vi "test图层-修改中.vi"() -> ()   [LabVIEW 2018]
doc: "This example demonstrates the use of binary morphological reconstruction in the particle analysis. The example allows you to keep the particles completely inside the ROI, completely outside the ROI or on the ROI."
uses:
  <vilib>/vision/NI_Vision_Development_Module.lvlib
panel:
  out "下":i32
  out "右":i32
  out "上":i32
  out "左":i32
  out "面积":i32
  out "标准差":sgl
  out "平均值":sgl
  out "最大灰度值":sgl
  out "最小灰度值":sgl
  out "选中框灰度表":u32[](graph)
  out "Image Dst Out":T1(plugin-control)
  out "全图灰度级信息":T2 {"标准差" format="%.2f"; "均值" format="%.2f"; "相邻灰度级间隔" format="%.2f"; "起始灰度值" format="%.2f"; "最大值" format="%.2f"; "最小值" format="%.2f"}
  out "图片灰度表":u32[](graph)
  in  "Font, Size & Style 2":T3={"Desired Font (Application)"=enum."Application Font", "[User-specified Font]"={"Font Name"="", "Size"=12, "Strikeout?"=FALSE, "Italic?"=FALSE, "Underline?"=FALSE, "Outline?"=FALSE, "Shadow?"=FALSE, "Bold?"=FALSE, "Rotation Angle"=0.0}, "Horizontal Alignment"=0, "Vertical Alignment"=0} {"Vertical Alignment" items=["Bottom", "Top", "Baseline"]; "Horizontal Alignment" items=["Left", "Center", "Right"]; "[User-specified Font]"."Rotation Angle" format="%.2f"}
  in  "选择框号":bool
  out "当前选择框的编号":dbl
  out "框总数":dbl
  in  "Font, Size & Style":T3={"Desired Font (Application)"=enum."Application Font", "[User-specified Font]"={"Font Name"="", "Size"=12, "Strikeout?"=FALSE, "Italic?"=FALSE, "Underline?"=FALSE, "Outline?"=FALSE, "Shadow?"=FALSE, "Bold?"=FALSE, "Rotation Angle"=0.0}, "Horizontal Alignment"=0, "Vertical Alignment"=0} {"Vertical Alignment" items=["Bottom", "Top", "Baseline"]; "Horizontal Alignment" items=["Left", "Center", "Right"]; "[User-specified Font]"."Rotation Angle" format="%.2f"}
  out "框组":T4(array[cluster])
  in  "单次删除":bool
  in  "Operation":enum16{"overlay rectangle"}(ring)
  out "标注图":T1(plugin-control)
  in  "退出标注":bool
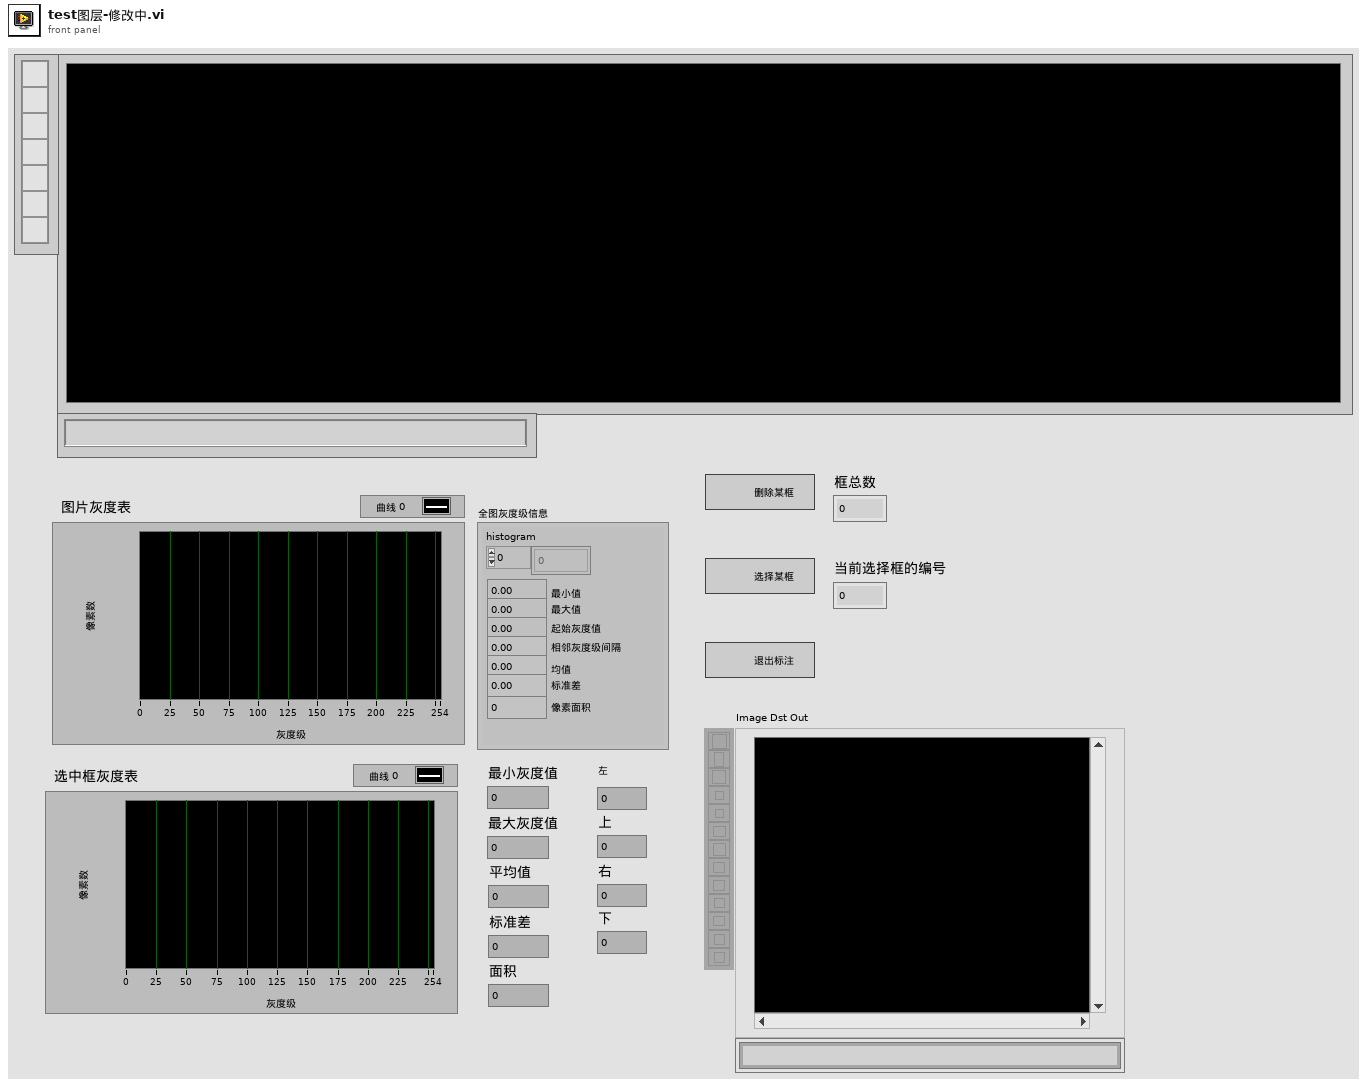
[diagram p1: front panel]
types:
  T1 = typedef "IMAQ Image.ctl" = refnum<image>
  T2 = cluster{"histogram":u32[], "最小值":sgl, "最大值":sgl, "起始灰度值":sgl, "相邻灰度级间隔":sgl, "均值":sgl, "标准差":sgl, "像素面积":i32}
  T3 = cluster{"Desired Font (Application)":enum16{"User-specified Font", "Application Font", "System Font", "Dialog Font"}, "[User-specified Font]":cluster{"Font Name":string, "Size":i16, "Strikeout?":bool, "Italic?":bool, "Underline?":bool, "Outline?":bool, "Shadow?":bool, "Bold?":bool, "Rotation Angle":dbl}, "Horizontal Alignment":i16, "Vertical Alignment":i16}
  T4 = cluster{"Global Rectangle":i32[], "Contours":cluster{"Contour Type":u32, "ROI Type":u32, "Points":i32[]}[]}[]
  T5 = typedef "Image Type" = u32
  T6 = cluster{"Global Rectangle":i32[], "Contours":cluster{"Contour Type":u32, "ROI Type":u32, "Points":i32[]}[]}
  T7 = typedef "IMAQ Rectangle" = cluster{"Left":i32, "Top":i32, "Right":i32, "Bottom":i32, "Rotation":dbl}
  T8 = cluster{"histogram":u32[], "Minimal Value":sgl, "Maximal Value":sgl, "Starting Value":sgl, "Interval Width":sgl, "Mean Value":sgl, "Standard  Variation":sgl, "Area (pixels)":i32}
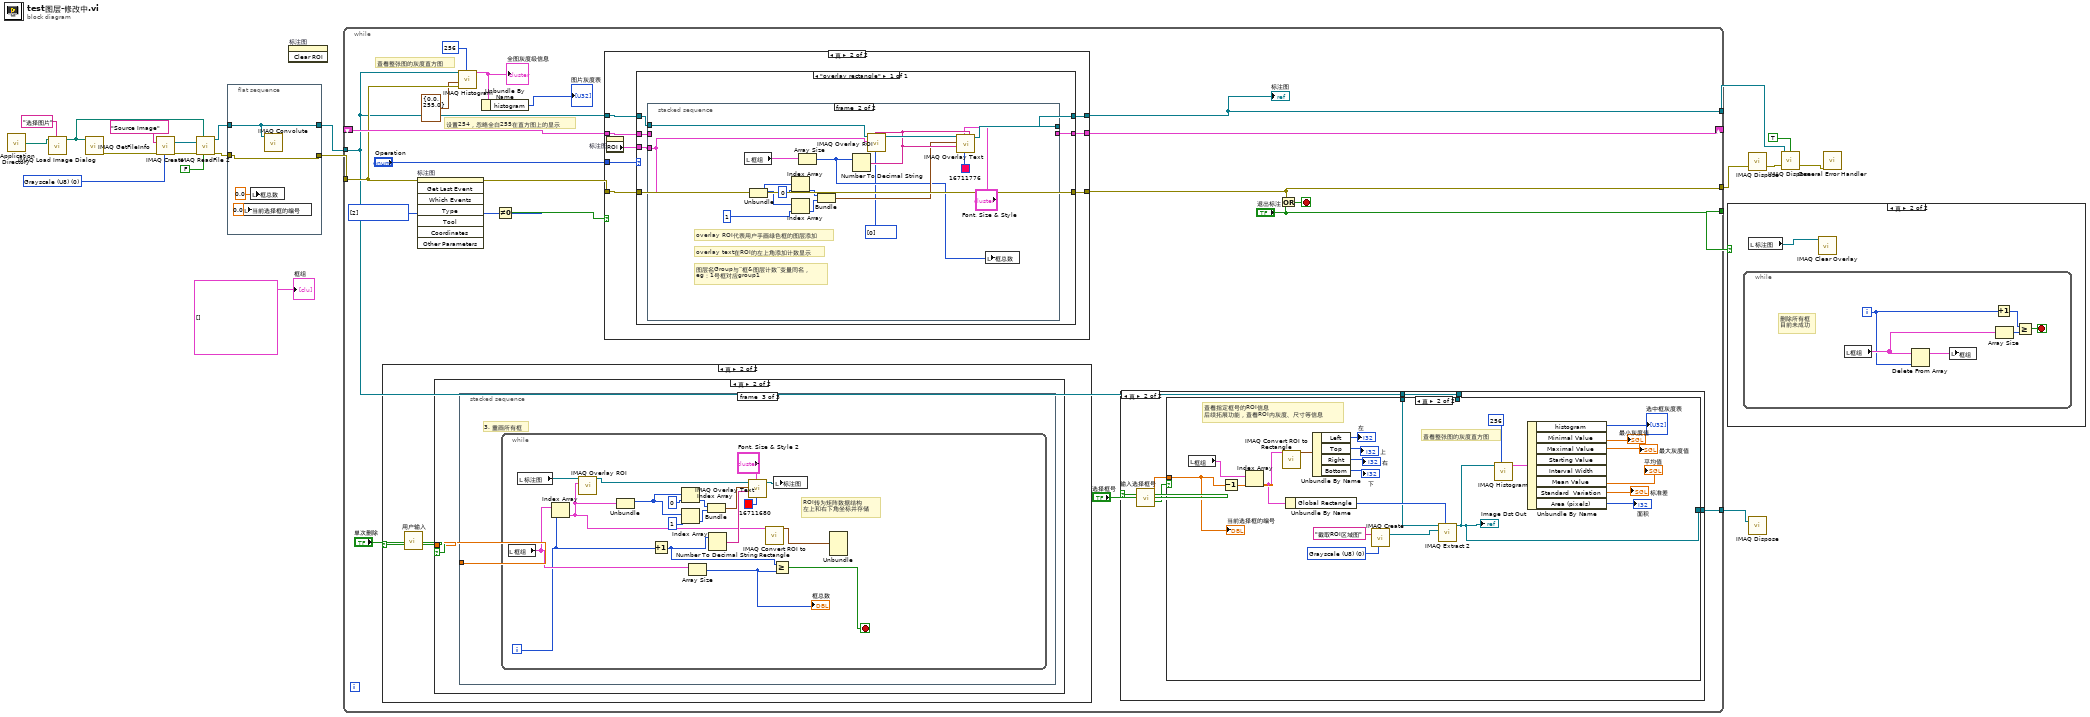
[diagram p0: block diagram]
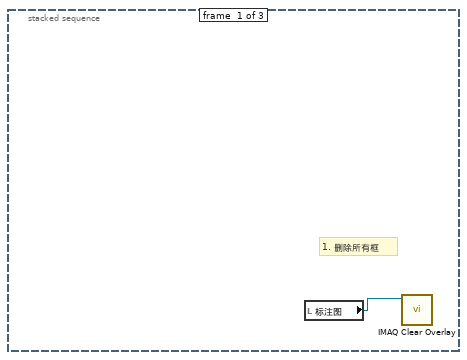
[diagram p7: hidden frame]
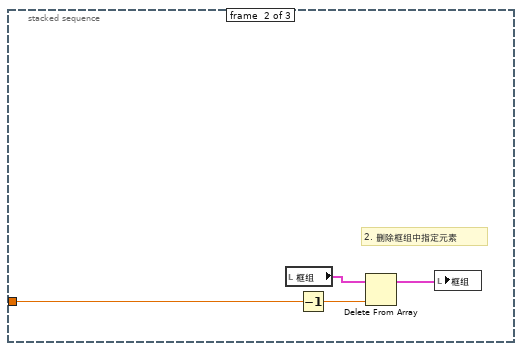
[diagram p8: hidden frame]
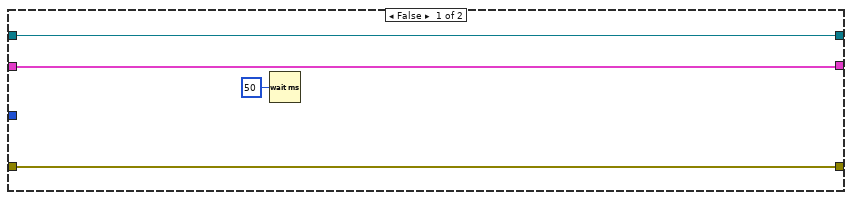
[diagram p9: hidden frame]
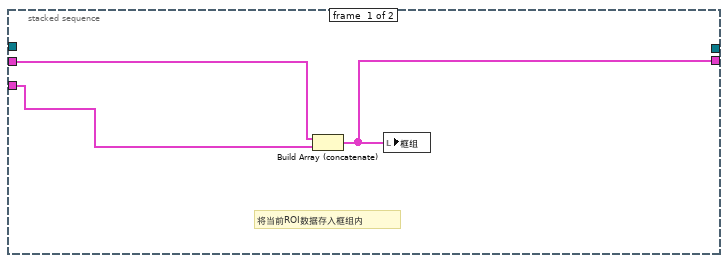
[diagram p10: hidden frame]
diagram:
  w12 = T5 0 items=["Grayscale (U8)", "Grayscale (I16)", "Grayscale (SGL)", "Complex (CSG)", "RGB (U32)", "HSL (U32)", "RGB (U64)", "Grayscale (U16)"] ("Image Type")
  n1 = call <vilib>:"Application Directory.vi"() -> ("Application Directory"=w13:path)
  n2 = call "IMAQ Load Image Dialog"("Prompt"="选择图片" ("prompt"), "Start Path"=w13) -> ("Path"=w19:path)  [unwired: 7 in, 2 out]
  n3 = call "IMAQ GetFileInfo"("File Path"=w19) -> ("error out"=w17:errorcluster)  [unwired: 4 in, 6 out]
  n4 = call "IMAQ Create"("Image Name"="Source Image", "Image Type"=w12, "error in (no error)"=w17) -> ("New Image"=w15:T1, "error out"=w14:errorcluster)  [unwired: 2 in]
  n5 = call "IMAQ ReadFile 2"("Use File Path Image Type"=FALSE, "File Path"=w19, "error in (no error)"=w14, "Image"=w15) -> ("error out"=w4:errorcluster, "Image Out"=w2:T1)  [unwired: 3 in, 3 out]
  n6 = flat-sequence {
    tunnel: [w23] -> w3
    tunnel: w4 -> [w23]
    tunnel: w2 -> [w22]
    tunnel: [w22] -> w1
    frame #0 {
      n7 = local write "当前选择框的编号"(0.0 ("当前框的编号")) -> ()
      n8 = local write "框总数"(0.0 ("框总数")) -> ()
      n9 = call "IMAQ Convolute"("Image Src"=w22) -> ()  [unwired: 9 in, 2 out]
    }
  }
  n10 = invoke on="标注图" class="ImageControl" method="Clear ROI"() -> ()  [unwired: 3 in, 3 out]
  n11 = while {
    tunnel: [w28] -> w10
    tunnel: [w41] -> w8
    shift-right: [w37] -> _
    shift-left: _ -> [w36]
    tunnel: ["退出标注"] -> w20
    tunnel: w3 -> [w33]
    tunnel: [w27] -> w5
    tunnel: w1 -> [w26]
    stop <- w40 stop-if-true
    w43 = i32[] [2] items=["No Event"=0, "Click Event"=1, "Draw Event"=2, "Size Event"=4, "Scroll Event"=5, "Double Click Event"=8] ("Which Events")
    # "设置254，忽略全白255在直方图上的显示"
    # "查看整张图的灰度直方图"
    n12 = case shown="真" "单次删除" {
      frame False {
      }
      frame True {
        n13 = call "用户输入"() -> ("框号"=w76:dbl, "确定"=w77:bool)  [unwired: 17 in, 1 out]
        n14 = case shown="真" w77 {
          tunnel: w76 -> [_ w78]
          frame False {
            # "用户取消操作"
          }
          frame True {
            n15 = stacked-sequence {
              tunnel: w78 -> [_ w82 _]
              frame #0 {
                # "1. 删除所有框"
                n16 = local read "标注图"() -> (w79:T1)
                n17 = call "IMAQ Clear Overlay"("Image"=w79) -> ()  [unwired: 9 in, 2 out]
              }
              frame #1 {
                # "2. 删除框组中指定元素"
                n18 = local read "框组"() -> (w83:T4)
                n19 = Decrement(x=w82) -> (x-1=w81:dbl)
                n20 = Delete From Array(array=w83, index=w81) -> (array with subset deleted=w80:T4)  [unwired: 1 in, 1 out]
                n21 = local write "框组"(w80) -> ()
              }
              frame #2 {
                # "3. 重画所有框"
                n22 = while {
                  i -> [w87]
                  stop <- w102 stop-if-true
                  # "ROI转为矩阵数据结构\n左上和右下角坐标并存储"
                  n23 = local read "框组"() -> (w95:T4)
                  n24 = local read "标注图"() -> (w101:T1)
                  n25 = Index Array(array=w95, index=w87) -> (element=w88:T6)
                  n26 = call "IMAQ Overlay ROI"("ROI Descriptor"=w88, "Image"=w101) -> ("Image Out"=w97:T1)  [unwired: 8 in, 1 out]
                  n27 = Unbundle(w88) -> ("Global Rectangle"=w91:i32[])  [unwired: 1 out]
                  n28 = Increment(x=w87) -> (x+1=w100:i32)
                  n29 = Index Array(array=w91, index=0 ("索引")) -> (element=w92:i32)
                  n30 = Index Array(array=w91, index=1 ("索引")) -> (element=w93:i32)
                  n31 = Array Size(array=w95) -> (size(s)=w85:i32)
                  "框总数" <- w85
                  n32 = Bundle(w92, w93) -> (w90:cluster{i32, i32})  [unwired: 1 in]
                  n33 = Number To Decimal String(number=w100) -> (decimal integer string=w98:string)  [unwired: 1 in]
                  n34 = call "IMAQ Overlay Text"("Text Color (black)"=u32 16711680, "Font, Size & Style"="Font, Size & Style 2", "String"=w98, "Origin"=w90, "Image"=w97) -> ("Image Out"=w96:T1)  [unwired: 5 in, 1 out]
                  n35 = call "IMAQ Convert ROI to Rectangle"("ROI Descriptor"=w88) -> ("Rectangle"=w86:T7)  [unwired: 8 in, 1 out]
                  n36 = Greater Or Equal?(x=w100, y=w85) -> (x >= y?=w102:bool)
                  n37 = local write "标注图"(w96) -> ()
                  n38 = Unbundle(w86) -> ()  [unwired: 5 out]
                }
              }
            }
          }
        }
      }
    }
    n39 = invoke on="标注图" class="ImageControl" method="Get Last Event"(error in=w33, "Which Events"=w43) -> (error out=w42:errorcluster, "Type"=w44:i32)  [unwired: 6 in, 6 out]
    n40 = call "IMAQ Histogram"("Number of Classes"=256, "error in (no error)"=w33, "Interval Range"=cluster{"Minimum":sgl, "Maximum":sgl} {"Minimum"=0.0, "Maximum"=255.0}, "Image"=w26) -> ("Histogram Report"=w30:T8)  [unwired: 6 in, 1 out]
    "全图灰度级信息" <- w30
    n41 = Unbundle By Name(w30) -> ("histogram"=→"图片灰度表":u32[])
    n42 = Not Equal To 0?(x=w44) -> (x != 0?=w38:bool)
    n43 = case shown="真" w38 {
      tunnel: w26 -> [w106 w114]
      tunnel: [w106 w113] -> w28
      tunnel: "Operation" -> [_ w111]
      tunnel: w42 -> [w105 w110]
      tunnel: [w105 w109] -> w41
      tunnel: [w103 w108] -> w37
      tunnel: w36 -> [w103 w107]
      frame False {
        n44 = Wait (ms)(milliseconds to wait=u32 50) -> ()  [unwired: 1 out]
      }
      frame True {
        n45 = property on="标注图" class="ImageControl"() -> ("ROI"=w112:T6)  [unwired: 2 in, 2 out]
        n46 = case shown="\"overlay rectangle\"" w111 {
          tunnel: w114 -> [w119]
          tunnel: w112 -> [w117]
          tunnel: [w118] -> w113
          tunnel: w110 -> [w120]
          tunnel: [w120] -> w109
          tunnel: [w116] -> w108
          tunnel: w107 -> [w115]
          frame "overlay rectangle" {
            n47 = stacked-sequence {
              tunnel: w119 -> [_ w130]
              tunnel: [_ w129] -> w118
              tunnel: w117 -> [w123 w126]
              tunnel: [w121 _] -> w116
              tunnel: w115 -> [w122 _]
              frame #0 {
                # "将当前ROI数据存入框组内"
                n48 = Build Array (concatenate)(w122, w123) -> (w121:T4)
                n49 = local write "框组"(w121) -> ()
              }
              frame #1 {
                # "图层名Group与“框&图层计数”变量同名，\neg：1号框对应group1"
                # "overlay text在ROI的左上角添加计数显示"
                # "overlay ROI代表用户手画绿色框的图层添加"
                n50 = local read "框组"() -> (w135:T4)
                n51 = Unbundle(w126) -> ("Global Rectangle"=w138:i32[])  [unwired: 1 out]
                n52 = Index Array(array=w138, index=0 ("索引")) -> (element=w137:i32)
                n53 = Index Array(array=w138, index=1 ("索引")) -> (element=w136:i32)
                n54 = Array Size(array=w135) -> (size(s)=w125:i32)
                n55 = Bundle(w137, w136) -> (w128:cluster{i32, i32})  [unwired: 1 in]
                n56 = Number To Decimal String(number=w125) -> (decimal integer string=w134:string)  [unwired: 1 in]
                n57 = call "IMAQ Overlay ROI"("Colors (Green)"=u32[] [0], "Group"=w134, "ROI Descriptor"=w126, "Image"=w130) -> ("Image Out"=w139:T1)  [unwired: 6 in, 1 out]
                n58 = call "IMAQ Overlay Text"("Group"=w134, "Text Color (black)"=u32 16711776, "Font, Size & Style"="Font, Size & Style", "String"=w134, "Origin"=w128, "Image"=w139) -> ("Image Out"=w129:T1)  [unwired: 4 in, 1 out]
                n59 = local write "框总数"(w125) -> ()
              }
            }
          }
        }
      }
    }
    "标注图" <- w28
    n60 = case shown="真" "选择框号" {
      tunnel: [w46 w49] -> w27
      tunnel: w26 -> [_ w48]
      tunnel: w26 -> [w46 w47]
      frame False {
      }
      frame True {
        n61 = call "输入选择框号"() -> ("框号"=w50:dbl, "确定"=w51:bool)  [unwired: 17 in, 1 out]
        n62 = case shown="真" w51 {
          tunnel: w50 -> [_ w74]
          tunnel: [w52 w63] -> w49
          tunnel: w48 -> [_ w67]
          tunnel: w47 -> [w52 _]
          frame False {
            # "用户取消操作"
          }
          frame True {
            w70 = T5 0 items=["Grayscale (U8)", "Grayscale (I16)", "Grayscale (SGL)", "Complex (CSG)", "RGB (U32)", "HSL (U32)", "RGB (U64)", "Grayscale (U16)"] ("Image Type")
            # "查看整张图的灰度直方图"
            # "查看指定框号的ROI信息\n后续拓展功能，查看ROI内灰度、尺寸等信息"
            n63 = local read "框组"() -> (w73:T4)
            n64 = Decrement(x=w74) -> (x-1=w75:dbl)
            n65 = Index Array(array=w73, index=w75) -> (element=w72:T6)
            n66 = call "IMAQ Convert ROI to Rectangle"("ROI Descriptor"=w72) -> ("Rectangle"=w57:T7)  [unwired: 8 in, 1 out]
            n67 = Unbundle By Name(w72) -> ("Global Rectangle"=w71:i32[])
            n68 = Unbundle By Name(w57) -> ("Left"=→"左":i32, "Top"=→"上":i32, "Right"=→"右":i32, "Bottom"=→"下":i32)
            n69 = call "IMAQ Create"("Image Name"="截取ROI区域图", "Image Type"=w70) -> ("New Image"=w68:T1)  [unwired: 3 in, 1 out]
            n70 = call "IMAQ Extract 2"("Optional Rectangle"=w71, "Image Dst"=w68, "Image Src"=w67) -> ("Image Dst Out"=w63:T1)  [unwired: 7 in, 1 out]
            "Image Dst Out" <- w63
            n71 = call "IMAQ Histogram"("Number of Classes"=256, "Image"=w63) -> ("Histogram Report"=w65:T8)  [unwired: 8 in, 1 out]
            n72 = Unbundle By Name(w65) -> ("histogram"=→"选中框灰度表":u32[], "Minimal Value"=→"最小灰度值":sgl, "Maximal Value"=→"最大灰度值":sgl, "Mean Value"=→"平均值":sgl, "Standard  Variation"=→"标准差":sgl, "Area (pixels)"=→"面积":i32)  [unwired: 2 out]
            "当前选择框的编号" <- w74
          }
        }
      }
    }
    n73 = Or(x=w41, y="退出标注") -> (x .or. y?=w40:bool)
  }
  n74 = case shown="真" w20 {
    frame False {
    }
    frame True {
      n75 = while {
        i -> [w145]
        stop <- w142 stop-if-true
        # "删除所有框\n目前未成功"
        n76 = local read "框组"() -> (w146:T4)
        n77 = Delete From Array(array=w146, index=w145) -> (array with subset deleted=w141:T4)  [unwired: 1 in, 1 out]
        n78 = local write "框组"(w141) -> ()
        n79 = Increment(x=w145) -> (x+1=w144:i32)
        n80 = Array Size(array=w146) -> (size(s)=w143:i32)
        n81 = Greater Or Equal?(x=w144, y=w143) -> (x >= y?=w142:bool)
      }
      n82 = local read "标注图"() -> (w140:T1)
      n83 = call "IMAQ Clear Overlay"("Image"=w140) -> ()  [unwired: 9 in, 2 out]
    }
  }
  n84 = call "IMAQ Dispose"("error in (no error)"=w8) -> ("error out"=w9:errorcluster)  [unwired: 2 in, 3 out]
  n85 = call "IMAQ Dispose"("Image"=w5) -> ()  [unwired: 2 in, 4 out]
  n86 = call "IMAQ Dispose"("All Images? (No)"=TRUE, "Image"=w10, "error in (no error)"=w9) -> ("error out"=w7:errorcluster)  [unwired: 3 out]
  n87 = call <vilib>:"General Error Handler.vi"("error in (no error)"=w7) -> ()  [unwired: 10 in, 5 out]
  "框组" <- T4 [] ("框组")
